vi "CalculateParameter.vi"(5 "波形解析正确":bool, 6 "enable":bool, 7 "PID 参数":T1={"proportional gain (Kc)"=1.0, "integral time (Ti, min)"=0.01, "derivative time (Td, min)"=0.0} {"derivative time (Td, min)" format="%.3f"; "integral time (Ti, min)" format="%.3f"; "proportional gain (Kc)" format="%.3f"}, 8 "采集的电信号值":dbl, 9 "插值后波形数组":dbl[](array[numeric])) -> (2 "输出相关参数":dbl, 3 "计算模块状态":bool)   [LabVIEW 2018]
uses:
  <vilib>/addons/control/pid/pid.llb/PID (DBL).vi
  <vilib>/addons/control/pid/NI_PID_pid.lvlib
panel:
  out "READY":bool
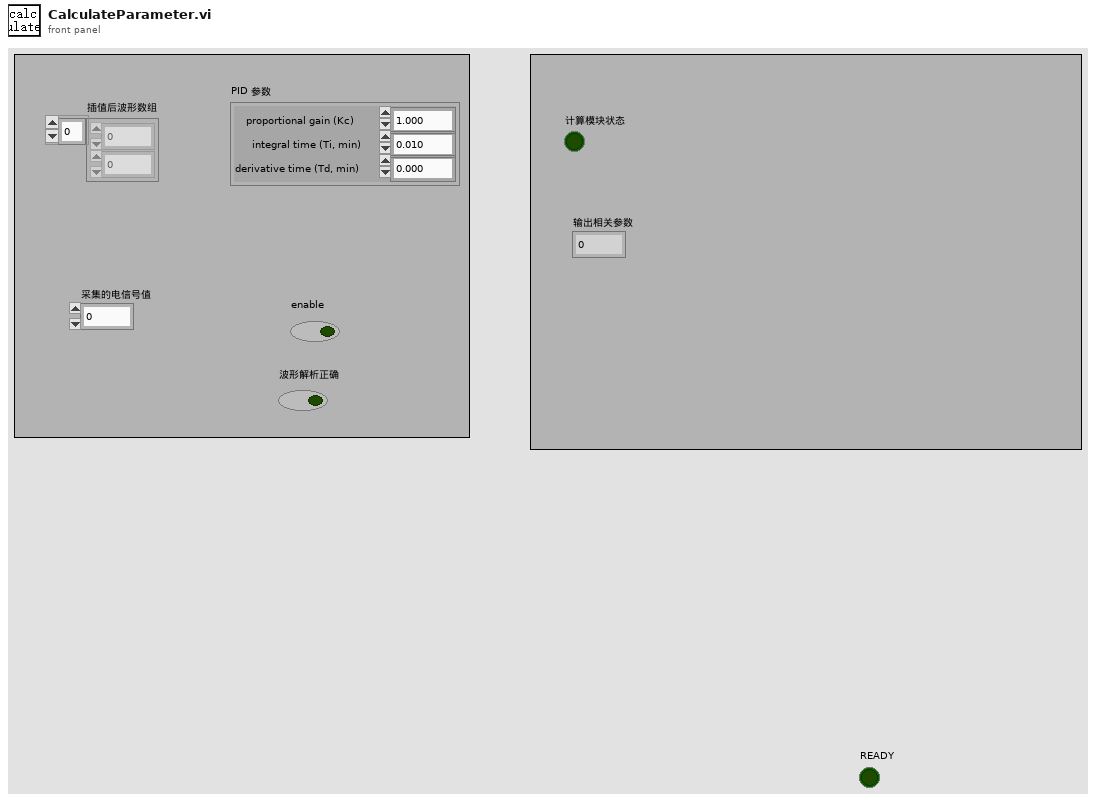
[diagram p1: front panel]
types:
  T1 = cluster{"proportional gain (Kc)":dbl, "integral time (Ti, min)":dbl, "derivative time (Td, min)":dbl}
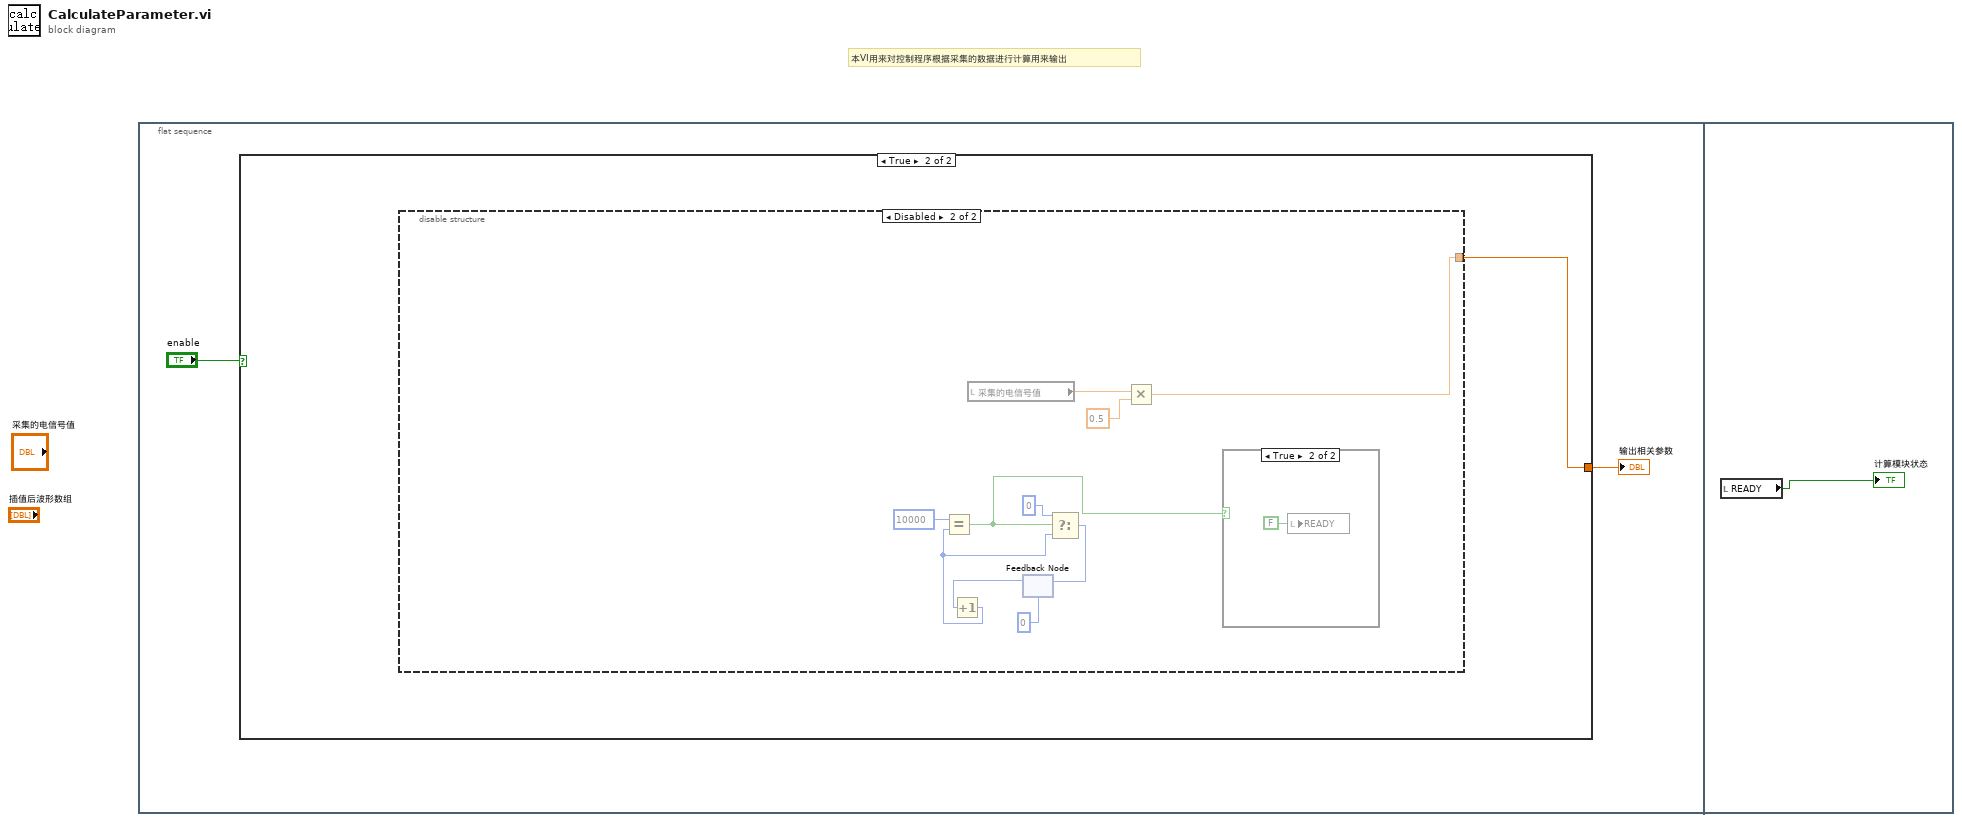
[diagram p0: block diagram]
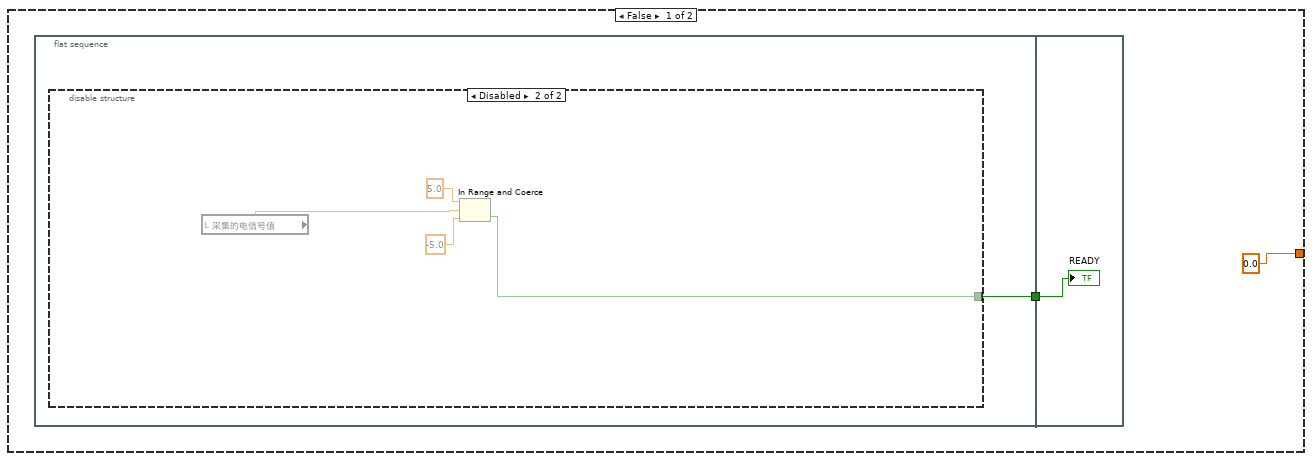
[diagram p2: hidden frame]
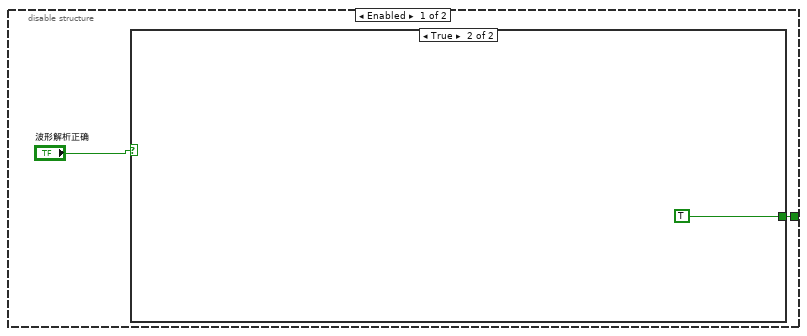
[diagram p3: hidden frame]
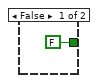
[diagram p4: hidden frame]
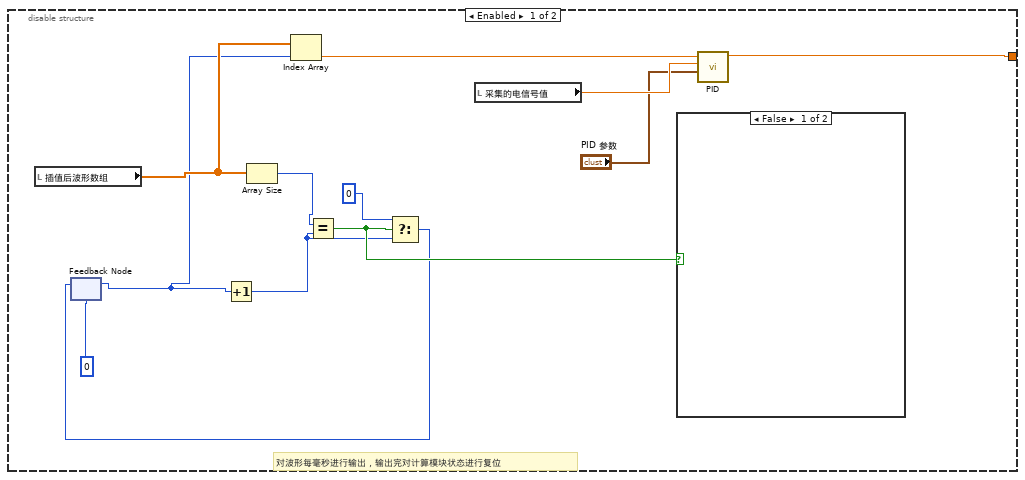
[diagram p5: hidden frame]
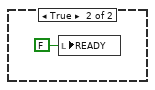
[diagram p6: hidden frame]
diagram:
  # "本VI用来对控制程序根据采集的数据进行计算用来输出"
  n1 = flat-sequence {
    frame #0 {
      n2 = case shown="True" "enable" {
        tunnel: [0.0 w15] -> w1
        frame False {
          n3 = flat-sequence {
            tunnel: [w5] -> w4
            tunnel: w4 -> [w14]
            frame #0 {
              n4 = disable-structure shown="Disabled" {
                disable-tunnel: [w7 w11] -> w5
                frame Enabled {
                  n5 = case shown="True" "波形解析正确" {
                    tunnel: [FALSE TRUE] -> w7
                    frame False {
                    }
                    frame True {
                    }
                  }
                }
                frame Disabled {
                  n6 = local read "采集的电信号值"() -> (w10:dbl)
                  n7 = In Range and Coerce(upper limit=5.0 ("上限"), x=w10, lower limit=-5.0 ("下限")) -> (In Range?=w11:bool)  [unwired: 1 out]
                }
              }
            }
            frame #1 {
              "READY" <- w14
            }
          }
        }
        frame True {
          n8 = disable-structure shown="Disabled" {
            disable-tunnel: [w16 w36] -> w15
            frame Enabled {
              # "对波形每毫秒进行输出，输出完对计算模块状态进行复位"
              n9 = local read "插值后波形数组"() -> (w25:dbl[])
              n10 = feedback #1(0) -> (w22:i32)
              n11 = Increment(x=w22) -> (x+1=w21:i32)
              n12 = Array Size(array=w25) -> (size(s)=w20:i32)
              n13 = Index Array(array=w25, index=w22) -> (element=w19:dbl)
              n14 = Equal?(x=w20, y=w21) -> (x = y?=w24:bool)
              n15 = Select(t=0, s=w24, f=w21) -> (s? t:f=w23:i32)
              n16 = feedback-in #1(w23) -> ()
              n17 = local read "采集的电信号值"() -> (w18:dbl)
              n18 = case shown="False" w24 {
                frame False {
                }
                frame True {
                  n19 = local write "READY"(FALSE ("READY")) -> ()
                }
              }
              n20 = call-poly <vilib>:"PID.vi"("PID gains"="PID 参数", "process variable"=w18, "setpoint"=w19) -> ("output"=w16:dbl)  [unwired: 7 in, 1 out]
            }
            frame Disabled {
              n21 = local read "采集的电信号值"() -> (w38:dbl)
              n22 = feedback #2(0) -> (w32:i32)
              n23 = Increment(x=w32) -> (x+1=w31:i32)
              n24 = Equal?(x=10000, y=w31) -> (x = y?=w29:bool)
              n25 = Select(t=0, s=w29, f=w31) -> (s? t:f=w33:i32)
              n26 = feedback-in #2(w33) -> ()
              n27 = Multiply(x=w38, y=0.5) -> (x*y=w36:dbl)
              n28 = case shown="True" w29 {
                frame False {
                }
                frame True {
                  n29 = local write "READY"(FALSE ("READY")) -> ()
                }
              }
            }
          }
        }
      }
      "输出相关参数" <- w1
    }
    frame #1 {
      n30 = local read "READY"() -> (→"计算模块状态":bool)
    }
  }
